vi "Global Variables.vi"() -> ()   [LabVIEW 2016]
panel:
  in  "Abort QA":bool
  in  "Popup to Display":string
  out "Display Popup":bool
  in  "Abort Scan":bool
  out "Timer Elapsed":bool
  out "Finished scanning?":bool
  in  "Pause Parallel DAQ":bool
  in  "Stop(QSM)":bool
  out "B-Field":dbl[](array[numeric])
  out "Graphing Array":dbl[][](array[numeric])
  # "These boolean globals are used to control various states of the QSM and should be written to sparingly."
  # "These variables only affect the popup (i.e. no user action) window, which displays a message to the user"
  # "These two array global variables are used ONLY for graphing and SHOULD NOT be used for any quantitative responses or reporting of results"
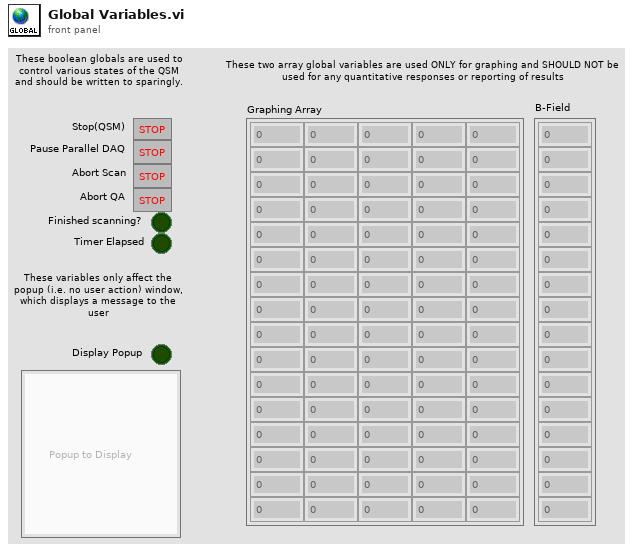
[diagram p1: front panel]
diagram:
